vi "Prompt for Step--UI Interlocks.vi"(8 "error in (no error)":errorcluster, 10 "Control Ref Map":map{string, refnum<vi>}(c390), 11 "Boolean Assertion in":refnum<class "Boolean Assertion.lvclass">) -> (0 "error out":errorcluster, 2 "Step Valid?":bool, 3 "Boolean Assertion out":refnum<class "Boolean Assertion.lvclass">)   [LabVIEW 2020, in "MacroAssert.lvlib" / "Boolean Assertion.lvclass"]
doc: "Enables or disables buttons within the \"Prompt for Step\" VI according to the current state of the system."
uses:
  Boolean Assertion.lvclass
  Assertion Step/Assertion Step.lvclass
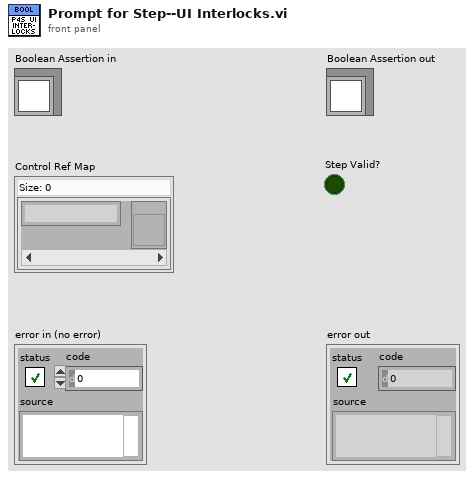
[diagram p1: front panel]
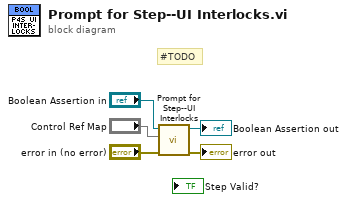
[diagram p0: block diagram]
diagram:
  # "#TODO"
  n1 = call-parent "Prompt for Step--UI Interlocks.vi"("error in (no error)"="error in (no error)", "Control Ref Map"="Control Ref Map", "Step in"="Boolean Assertion in") -> ("error out"=→"error out":errorcluster, "Step out"=→"Boolean Assertion out":refnum<class "Boolean Assertion.lvclass">)  [unwired: 6 in, 1 out]
